vi "Self Test.vi"(8 "error in (no error)":errorcluster, 11 "VISA resource name":refnum<visa-resource-name>) -> (0 "error out":errorcluster, 1 "self-test response":string, 2 "self-test error":bool, 3 "VISA resource name out":refnum<visa-resource-name>)   [LabVIEW 2020, in "Agilent E364X Series.lvlib"]
doc: "This VI causes the instrument to perform a self-test and returns the results. A boolean indicates if the instrument passed self-test, and string contains the instruments response."
uses:
  Agilent E364X Series.lvlib
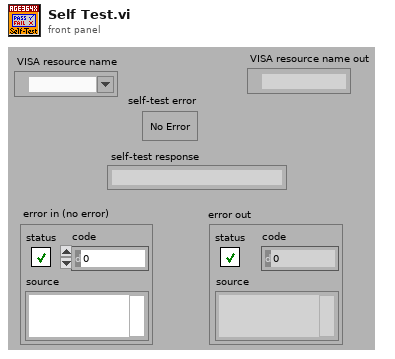
[diagram p1: front panel]
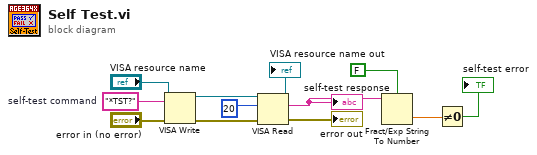
[diagram p0: block diagram]
diagram:
  w12 = "*TST?"  # self-test command
  n1 = VISA Write(VISA resource name="VISA resource name", write buffer=w12, error in (no error)="error in (no error)") -> (VISA resource name out=w4:refnum<visa-resource-name>, error out=w7:errorcluster)  [unwired: 1 out]
  n2 = VISA Read(VISA resource name=w4, byte count=u32 20, error in (no error)=w7) -> (VISA resource name out=→"VISA resource name out":refnum<visa-resource-name>, read buffer=w9:string, error out=→"error out":errorcluster)  [unwired: 1 out]
  "self-test response" <- w9
  n3 = Fract/Exp String To Number(use system decimal point (T)=FALSE, string=w9) -> (number=w3:dbl)  [unwired: 2 in, 1 out]
  n4 = Not Equal To 0?(x=w3) -> (x != 0?=→"self-test error":bool)
